vi "ProdaNG.Tree.Proc.GetTag.vi"(7 "Tree":refnum<vi>, 11 "Tag":string) -> (0 "parent":bool, 1 "Process Found":bool, 2 "Identification":T1, 3 "ProfInfo":string[](array[string]), 4 "SlotNo":i32)   [LabVIEW 2016]
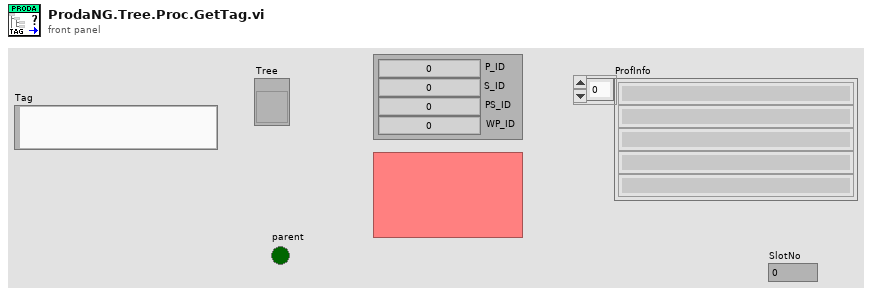
[diagram p1: front panel]
types:
  T1 = cluster{"P_ID":i32, "S_ID":i32, "PS_ID":i32, "WP_ID":i32}
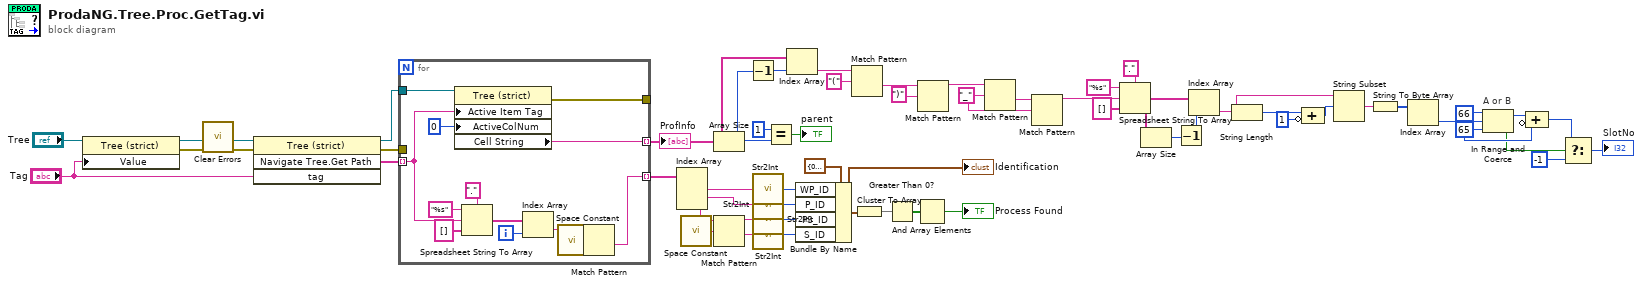
[diagram p0: block diagram]
diagram:
  w9 = "_" ("regular expression")
  w16 = 65 ("lower limit")
  # "A or B"
  n1 = property on="Property Node" class="Tree (strict)"(reference="Tree", "Value"="Tag") -> (reference out=w35:refnum<vi>, error out=w34:errorcluster)  [unwired: 1 in]
  n2 = call <vilib>:"Clear Errors.vi"("error in (no error)"=w34) -> ("error out"=w33:errorcluster)  [unwired: 5 in, 1 out]
  n3 = invoke on="Invoke Node" class="Tree (strict)" method="Navigate Tree.Get Path"(reference=w35, error in=w33, "tag"="Tag") -> (reference out=w42:refnum<vi>, error out=w37:errorcluster, "Navigate Tree:Get Path"=w45:string[])  [unwired: 1 in, 1 out]
  n4 = for {
    tunnel: w45 -> [w60] mode=indexing
    tunnel: [w58] -> w57 mode=indexing
    tunnel: [w69] -> w29 mode=indexing
    tunnel: [w68] -> _
    tunnel: w42 -> [w66]
    tunnel: w37 -> [_]
    i -> [w61]
    n5 = property on="Property Node" class="Tree (strict)"(reference=w66, "Active Item Tag"=w60, "ActiveColNum"=0 ("Active Cell:Active Column Number")) -> (error out=w68:errorcluster, "Cell String"=w69:string)  [unwired: 1 in, 1 out]
    n6 = Spreadsheet String To Array(delimiter (Tab)=".", format string="%s", spreadsheet string=w60, array type (2D Dbl)=string[] []) -> (array=w62:string[])
    n7 = Index Array(array=w62, index=w61) -> (element=w59:string)
    n8 = call <vilib>:"Space Constant.vi"() -> ("String"=w70:string)
    n9 = Match Pattern(string=w59, regular expression=w70) -> (after substring=w58:string)  [unwired: 1 in, 3 out]
  }
  "ProfInfo" <- w29
  n10 = Index Array(array=w57) -> (element #1=w56:string, element #2=w51:string, element #3=w43:string)  [unwired: 3 in]
  n11 = call <vilib>:"Space Constant.vi"() -> ("String"=w55:string)
  n12 = Array Size(array=w29) -> (size(s)=w31:i32)
  n13 = Match Pattern(string=w43, regular expression=w55) -> (before substring=w54:string, after substring=w48:string)  [unwired: 1 in, 2 out]
  n14 = Decrement(x=w31) -> (x-1=w30:i32)
  n15 = call "Str2Int.vi"("string"=w56) -> ("Numeric"=w53:i32)
  n16 = call "Str2Int.vi"("string"=w51) -> ("Numeric"=w52:i32)
  n17 = call "Str2Int.vi"("string"=w54) -> ("Numeric"=w50:i32)
  n18 = call "Str2Int.vi"("string"=w48) -> ("Numeric"=w49:i32)
  n19 = Equal?(x=1, y=w31) -> (x = y?=→"parent":bool)
  n20 = Index Array(array=w29, index=w30) -> (element=w28:string)
  n21 = Bundle By Name(cluster=T1 {"P_ID"=0, "S_ID"=0, "PS_ID"=0, "WP_ID"=0} ("Identification"), "WP_ID"=w53, "P_ID"=w52, "PS_ID"=w50, "S_ID"=w49) -> (w40:T1)
  "Identification" <- w40
  n22 = Match Pattern(string=w28, regular expression="(") -> (after substring=w26:string)  [unwired: 1 in, 3 out]
  n23 = Cluster To Array(cluster=w40) -> (array=w47:i32[])
  n24 = Greater Than 0?(x=w47) -> (x > 0?=w46:bool[])
  n25 = And Array Elements(Boolean array=w46) -> (logical AND=→"Process Found":bool)
  n26 = Match Pattern(string=w26, regular expression=")") -> (before substring=w10:string)  [unwired: 1 in, 3 out]
  n27 = Match Pattern(string=w10, regular expression=w9) -> (after substring=w11:string)  [unwired: 1 in, 3 out]
  n28 = Match Pattern(string=w11, regular expression=w9) -> (before substring=w5:string)  [unwired: 1 in, 3 out]
  n29 = Spreadsheet String To Array(delimiter (Tab)=".", format string="%s", spreadsheet string=w5, array type (2D Dbl)=string[] []) -> (array=w3:string[])
  n30 = Array Size(array=w3) -> (size(s)=w4:i32)
  n31 = Decrement(x=w4) -> (x-1=w2:i32)
  n32 = Index Array(array=w3, index=w2) -> (element=w1:string)
  n33 = String Length(string=w1) -> (length=w24:i32)
  n34 = Compound Arithmetic op=ADD(w24, invert 1 ("value")) -> (w21:i32)
  n35 = String Subset(string=w1, offset (0)=w21) -> (substring=w22:string)  [unwired: 1 in]
  n36 = String To Byte Array(string=w22) -> (unsigned byte array=w20:u8[])
  n37 = Index Array(array=w20) -> (element=w19:u8)  [unwired: 1 in]
  n38 = In Range and Coerce(upper limit=66 ("lower limit"), x=w19, lower limit=w16) -> (coerced(x)=w17:i32, In Range?=w15:bool)
  n39 = Compound Arithmetic op=ADD(w17, invert w16) -> (w14:i32)
  n40 = Select(t=w14, s=w15, f=-1) -> (s? t:f=→"SlotNo":i32)
